vi "Cache.Find.vi"(7 "Idx":i32, 8 "error in (no error)":errorcluster, 9 "Serial":string, 10 "Variant":string, 11 "Data in":T7) -> (0 "error out":errorcluster, 1 "ProductComponent":T1, 2 "Result":T2, 3 "Data out":T7)   [LabVIEW 2016]
uses:
  Cache.Data.ctl
  Cache.Data.Status.ctl
  Cache.Data.Sets.ctl
  Cache.TestSteps.Fglb.ResultData.ctl
  Database/ProdaNG/Controls/ProdaNG.ProcessResult.ctl
  Database/ProdaNG/Controls/ProdaNG.ProcessStepResult.ctl
  Database/ProdaNG/Controls/ProdaNG.TestStepResult.ctl
  Database/ProdaNG/Controls/ProdaNG.TestValueResult.ctl
  Database/ProdaNG/Controls/ProdaNG.ProductComponent.ctl
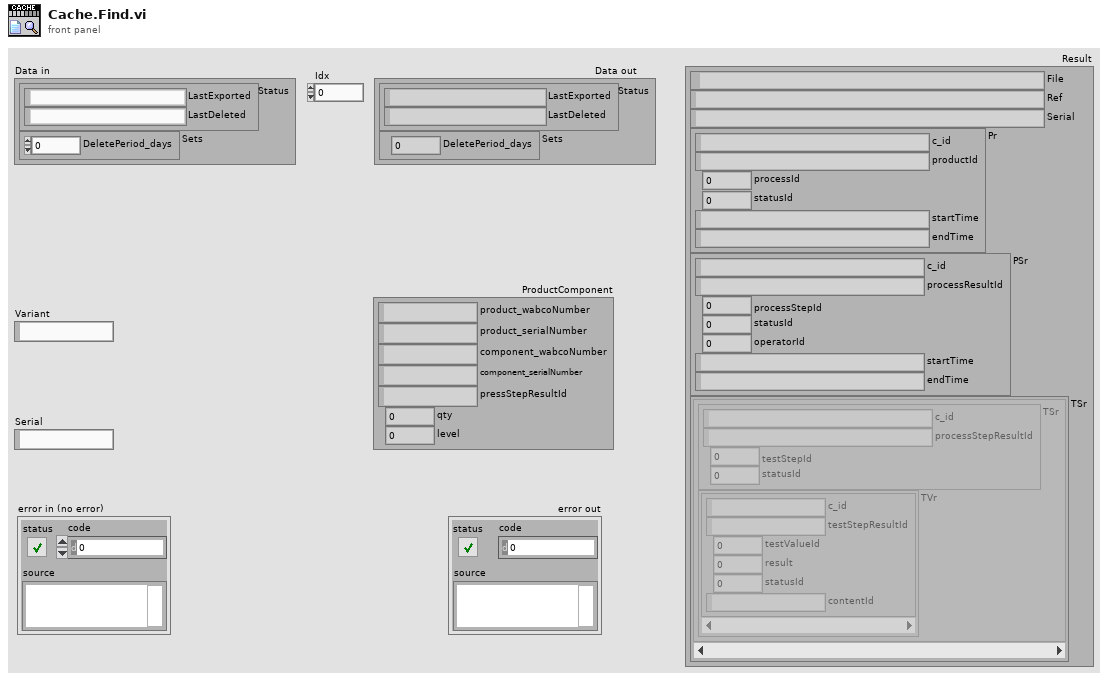
[diagram p1: front panel]
types:
  T1 = typedef "ProdaNG.ProductComponent.ctl" = cluster{"product_wabcoNumber":string, "product_serialNumber":string, "component_wabcoNumber":string, "component_serialNumber":string, "pressStepResultId":string, "qty":i32, "level":i32}
  T2 = typedef "Cache.TestSteps.Fglb.ResultData.ctl" = cluster{"File":path, "Ref":string, "Serial":string, "Pr":T3, "PSr":T4, "TSr":cluster{"TSr":T5, "TVr":T6[]}[]}
  T3 = typedef "ProdaNG.ProcessResult.ctl" = cluster{"c_id":string, "productId":string, "processId":i32, "statusId":i32, "startTime":string, "endTime":string}
  T4 = typedef "ProdaNG.ProcessStepResult.ctl" = cluster{"c_id":string, "processResultId":string, "processStepId":i32, "statusId":i32, "operatorId":i32, "startTime":string, "endTime":string}
  T5 = typedef "ProdaNG.TestStepResult.ctl" = cluster{"c_id":string, "processStepResultId":string, "testStepId":i32, "statusId":i32}
  T6 = typedef "ProdaNG.TestValueResult.ctl" = cluster{"c_id":string, "testStepResultId":string, "testValueId":i32, "result":dbl, "statusId":i32, "contentId":string}
  T7 = typedef "Cache.Data.ctl" = cluster{"Status":T8, "Sets":T9}
  T8 = typedef "Cache.Data.Status.ctl" = cluster{"LastExported":string, "LastDeleted":string}
  T9 = typedef "Cache.Data.Sets.ctl" = cluster{"DeletePeriod_days":dbl}
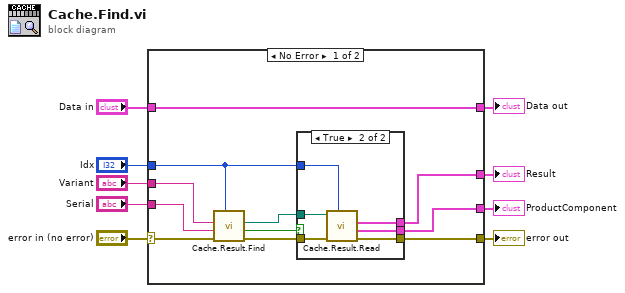
[diagram p0: block diagram]
diagram:
  n1 = case shown="No Error" "error in (no error)" {
    selector: "error in (no error)" -> [w17 w29]
    tunnel: "Idx" -> [w15 _]
    tunnel: [w20 w29] -> w8
    tunnel: "Data in" -> [w10 w28]
    tunnel: [w10 w28] -> w5
    tunnel: [w19 _] -> w4
    tunnel: [w18 _] -> w3
    tunnel: "Serial" -> [w14 _]
    tunnel: "Variant" -> [w13 _]
    frame No Error {
      n2 = call "Cache.Result.Find.vi"("Idx"=w15, "error in (no error)"=w17, "Serial"=w14, "Variant"=w13) -> ("error out"=w16:errorcluster, "Found?"=w12:bool, "File"=w11:path)  [unwired: 5 in]
      n3 = case shown="True" w12 {
        tunnel: [w21 w27] -> w20
        tunnel: [_ w26] -> w19
        tunnel: [_ w25] -> w18
        tunnel: w16 -> [w21 w24]
        tunnel: w15 -> [_ w23]
        tunnel: w11 -> [_ w22]
        frame False {
        }
        frame True {
          n4 = call "Cache.Result.Read.vi"("Idx"=w23, "error in (no error)"=w24, "ResultsPath"=w22) -> ("error out"=w27:errorcluster, "ProductComponent"=w25:T1, "Result"=w26:T2)  [unwired: 6 in]
        }
      }
    }
    frame Error {
    }
  }
  "error out" <- w8
  "Data out" <- w5
  "Result" <- w4
  "ProductComponent" <- w3
